vi "Set Config Values.vi"(8 "error in (no error)":errorcluster, 11 "Coins":cluster{"Boolean Text":string, "Value":dbl}[](array[cluster])) -> (0 "error out":errorcluster)   [LabVIEW 2020, in "Config.lvlib"]
uses:
  Config.lvlib
  <vilib>/Utility/xml.llb/Write to XML File(string).vi
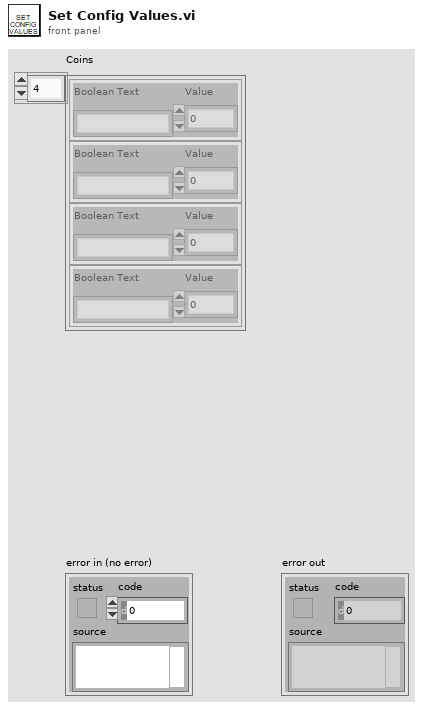
[diagram p1: front panel]
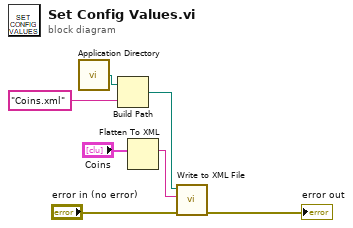
[diagram p0: block diagram]
diagram:
  n1 = call <vilib>:"Application Directory.vi"() -> ("Application Directory"=w7:path)
  n2 = Build Path(base path=w7, name or relative path="Coins.xml") -> (appended path=w6:path)
  n3 = Flatten To XML(6:"Coins") -> (2:w1:string)
  n4 = call-poly <vilib>:"Write to XML File.vi"("error in (no error)"="error in (no error)", "XML Input"=w1, "XML File Path"=w6) -> ("error out"=→"error out":errorcluster)  [unwired: 6 in, 2 out]
